vi "Aggregated var speed Test 2.vi"() -> ()   [LabVIEW 2021]
uses:
  <vilib>/TSA/Abstract Data Classes/Abs_Types/Double Float/Support/Type.ctl
  Source/Omni-Bus/Omni_Bus.lvclass
  Source/Aggregator Bus/Aggregator Bus.lvclass
  C:/Users/Tim/Documents/GitHub/Omni-Bus/Source/Omni-Bus/Bus Access/Bus_Access.lvclass
  Source/Omni-Bus/Support/Broad Types.ctl
  <vilib>/TSA/Abstract Data Classes/Abs_Types/Type/Abs_Type.lvclass
  Source/Omni-Bus/Bus Access/Bus_Access.lvclass/Bus_Access.ctl
  Source/Omni-Bus/Bus Access/Properties/Write Tags.vi
  Source/Omni-Bus/Bus Access/Properties/Write Values.vi
  <vilib>/TSA/Abstract Data Classes/Abs_Types/Boolean/Abs_Boolean.lvclass
  C:/Program Files (x86)/National Instruments/LabVIEW 2021/vi.lib/TSA/Abstract Data Classes/Abs_Types/Type/Abs_Type.lvclass
  <vilib>/TSA/Abstract Data Classes/Constants/Support/DBL/Const_DBL.lvclass
  <vilib>/TSA/Abstract Data Classes/Abs_Types/String/Abs_String.lvclass
  <vilib>/TSA/Abstract Data Classes/Abs_Types/I32 Integer/Abs_I32 Integer.lvclass
  <vilib>/TSA/Abstract Data Classes/Constants/Support/Bool/Bool.vi
  <vilib>/TSA/Abstract Data Classes/Constants/Support/DBL/DBL.vi
  <vilib>/TSA/Abstract Data Classes/Constants/Support/Str/Str.vi
  <vilib>/TSA/Abstract Data Classes/Constants/Support/I32/I32.vi
  <vilib>/TSA/Abstract Data Classes/Abs_Types/Double Float/Abs_Double Float.lvclass
  <vilib>/TSA/Abstract Data Classes/Constants/Support/Str/Const_Str.lvclass
  <vilib>/TSA/Abstract Data Classes/Constants/Support/Bool/Const_Bool.lvclass
  <vilib>/TSA/Abstract Data Classes/Constants/Support/I32/Const_I32.lvclass
panel:
  out "error out":errorcluster
  out "x-y":dbl
  out "Value":T1
  out "Tags":string[](array[string])
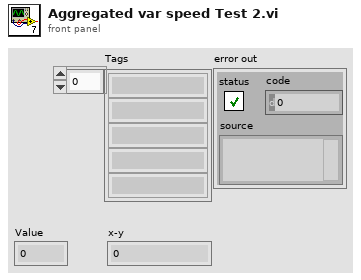
[diagram p1: front panel]
types:
  T1 = typedef "Abs_Double Float.lvclass/Type.ctl" = dbl
  T2 = typedef "Omni_Bus.lvclass/Broad Types.ctl" = enum16{"All Tags", "NI Specific Type", "Boolean", "String", "Numeric", "Float", "Integer", "Collection", "All Value Types", "Non Value Types"}
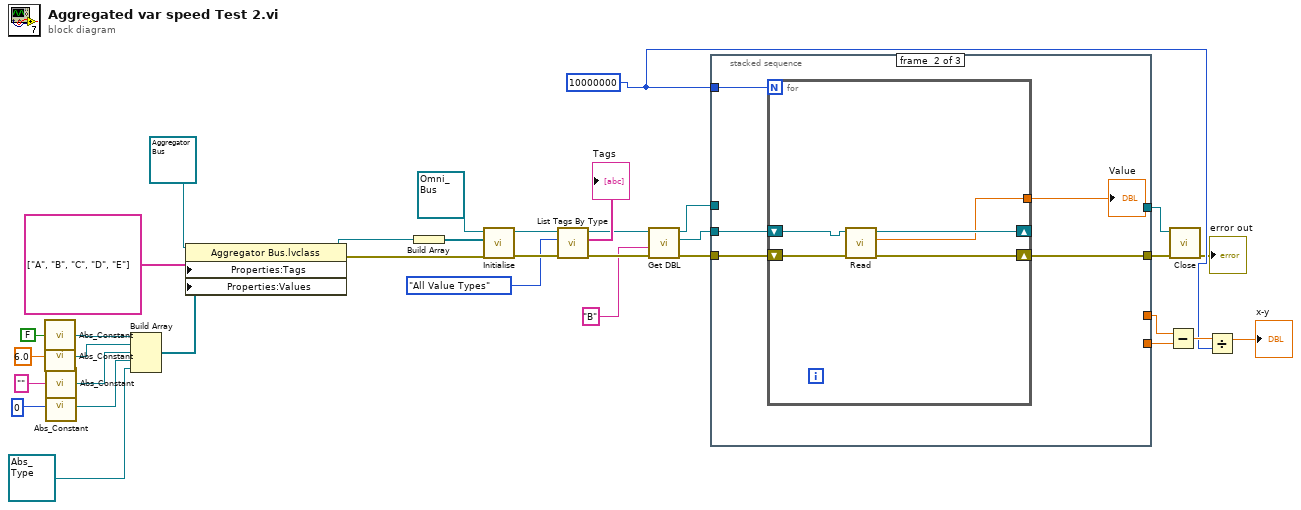
[diagram p0: block diagram]
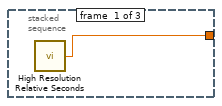
[diagram p2: hidden frame]
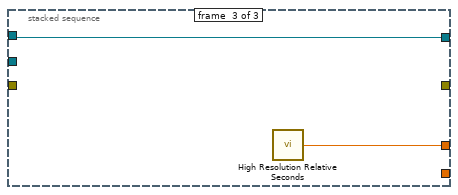
[diagram p3: hidden frame]
diagram:
  w10 = 10000000
  n1 = call-poly <vilib>:"Abs_Constant.vi"("Boolean"=FALSE) -> ("Abs_Boolean.lvclass"=w28:refnum<class "Abs_Boolean.lvclass">)  [unwired: 4 in]
  n2 = call-poly <vilib>:"Abs_Constant.vi"("Value"=6.0) -> ("Constant"=w27:refnum<class "Const_DBL.lvclass">)  [unwired: 4 in]
  n3 = call-poly <vilib>:"Abs_Constant.vi"("String"="") -> ("Abs_String.lvclass"=w26:refnum<class "Abs_String.lvclass">)  [unwired: 4 in]
  n4 = call-poly <vilib>:"Abs_Constant.vi"("Value"=0) -> ("Constant"=w18:refnum<class "Abs_I32 Integer.lvclass">)  [unwired: 4 in]
  n5 = Build Array(w28, w27, w26, w18, refnum<class "Abs_Type.lvclass"> refnum ("Abs_Type.lvclass")) -> (w23:refnum<class "Abs_Type.lvclass">[])
  n6 = property class="Aggregator Bus.lvclass"(reference=refnum<class "Aggregator Bus.lvclass"> refnum ("Data in"), "Properties:Tags"=string[] ["A", "B", "C", "D", "E"] ("Tags"), "Properties:Values"=w23) -> (reference out=w31:refnum<class "Aggregator Bus.lvclass">, error out=w32:errorcluster)  [unwired: 1 in]
  n7 = Build Array(w31) -> (w33:refnum<class "Aggregator Bus.lvclass">[])
  n8 = call-dynamic "Initialise.vi"("error in (no error)"=w32, "Bus Access"=w33, "Var Bus in"=refnum<class "Omni_Bus.lvclass"> refnum) -> ("error out"=w21:errorcluster, "Var Bus out"=w22:refnum<class "Omni_Bus.lvclass">)  [unwired: 7 in]
  n9 = call-dynamic "List Tags By Type.vi"("error in (no error)"=w21, "Broad Types"=Broad_Types."All Value Types", "Var Bus in"=w22) -> ("error out"=w6:errorcluster, "Tags"=→"Tags":string[], "Var Bus out"=w7:refnum<class "Omni_Bus.lvclass">)  [unwired: 5 in, 1 out]
  n10 = call-dynamic "Get DBL.vi"("error in (no error)"=w6, "Tag"="B", "Var Bus in"=w7) -> ("error out"=w3:errorcluster, "Value Out"=w4:refnum<class "Abs_Double Float.lvclass">, "Var Bus out"=w2:refnum<class "Omni_Bus.lvclass">)  [unwired: 6 in]
  n11 = stacked-sequence {
    tunnel: w4 -> [_ w38 _]
    tunnel: w3 -> [_ w37 _]
    tunnel: [_ _ w46] -> w15
    tunnel: [_ _ w47] -> w14
    tunnel: [w35 _ _] -> w13
    tunnel: w10 -> [_ w39 _]
    tunnel: w2 -> [_ _ w46]
    tunnel: [_ w36 _] -> w1
    frame #0 {
      n12 = call <vilib>:"High Resolution Relative Seconds.vi"() -> ("relative seconds"=w35:dbl)
    }
    frame #1 {
      n13 = for {
        N: w39 -> [_]
        shift-right: [w44] -> _
        shift-left: w38 -> [w45]
        tunnel: [w43] -> w40
        shift-right: [w41] -> w36
        shift-left: w37 -> [w42]
        n14 = call-dynamic "Read.vi"("error in (no error)"=w42, "Double Float.lvclass_340760 in"=w45) -> ("error out"=w41:errorcluster, "Value"=w43:T1, "Double Float.lvclass_340760 out"=w44:refnum<class "Abs_Double Float.lvclass">)  [unwired: 7 in]
      }
      "Value" <- w40
    }
    frame #2 {
      n15 = call <vilib>:"High Resolution Relative Seconds.vi"() -> ("relative seconds"=w47:dbl)
    }
  }
  n16 = Subtract(x=w14, y=w13) -> (x-y=w12:dbl)
  n17 = call-dynamic "Close.vi"("error in (no error)"=w1, "Data in"=w15) -> ("error out"=→"error out":errorcluster)  [unwired: 8 in, 1 out]
  n18 = Divide(x=w12, y=w10) -> (x/y=→"x-y":dbl)
